vi "Data_taker_ver2.1.vi"() -> ()   [LabVIEW 2021]
uses:
  <vilib>/express/express analysis/Spectral/Block/exnSpectralBlock spectral measurements power poly.vi
  <vilib>/express/express analysis/Spectral/Block/exnSpectralBlock spectral measurements power DDT.vi
  <userlib>/SMC100 Controller_Drivers/SMC100.llb/enter / leave disable state.vi
  <vilib>/express/express analysis/Spectral/Block/exnSpectralBlock spectral measurements power WFM.vi
  <vilib>/express/express analysis/Spectral/XNode/ExpressSpectralMeasurementsBlockNode.xnode
panel:
  out "Loop count":i32
  in  "Averaging":bool
  out "Spectrum":cluster{"x axis":dbl[], "y data":dbl[]}(graph)
  out "Average intensity":cluster{"x axis":dbl[], "y data":dbl[]}(graph)
  out "Intensity (cut)":dynamicdata(graph)
  out "Spectrum":dynamicdata(graph)
  out "Intensity (raw)":dynamicdata(graph)
  in  "Repeat":i32
  out "Status":string
  in  "Begin Offset":dbl=1.0
  in  "Spectrum data path":path
  in  "Intensity data path":path
  in  "Velocity value (mm/s)":dbl
  in  "number of samples":i32=20000
  in  "rate":dbl=1000.0
  out "total time":dbl
  out "Displacement (mm)":dbl
  out "VISA Handle in":refnum<visa-resource-name>
  in  "unlock ?":bool
  in  "Unlock":bool
  out "Now position (mm)":dbl
  in  "Current absolute position":bool
  in  "Stop whole program":bool
  in  "Stop moving":bool
  in  "Start up/Reset":bool
  in  "Initialize":bool
  in  "Move  + data taking":bool
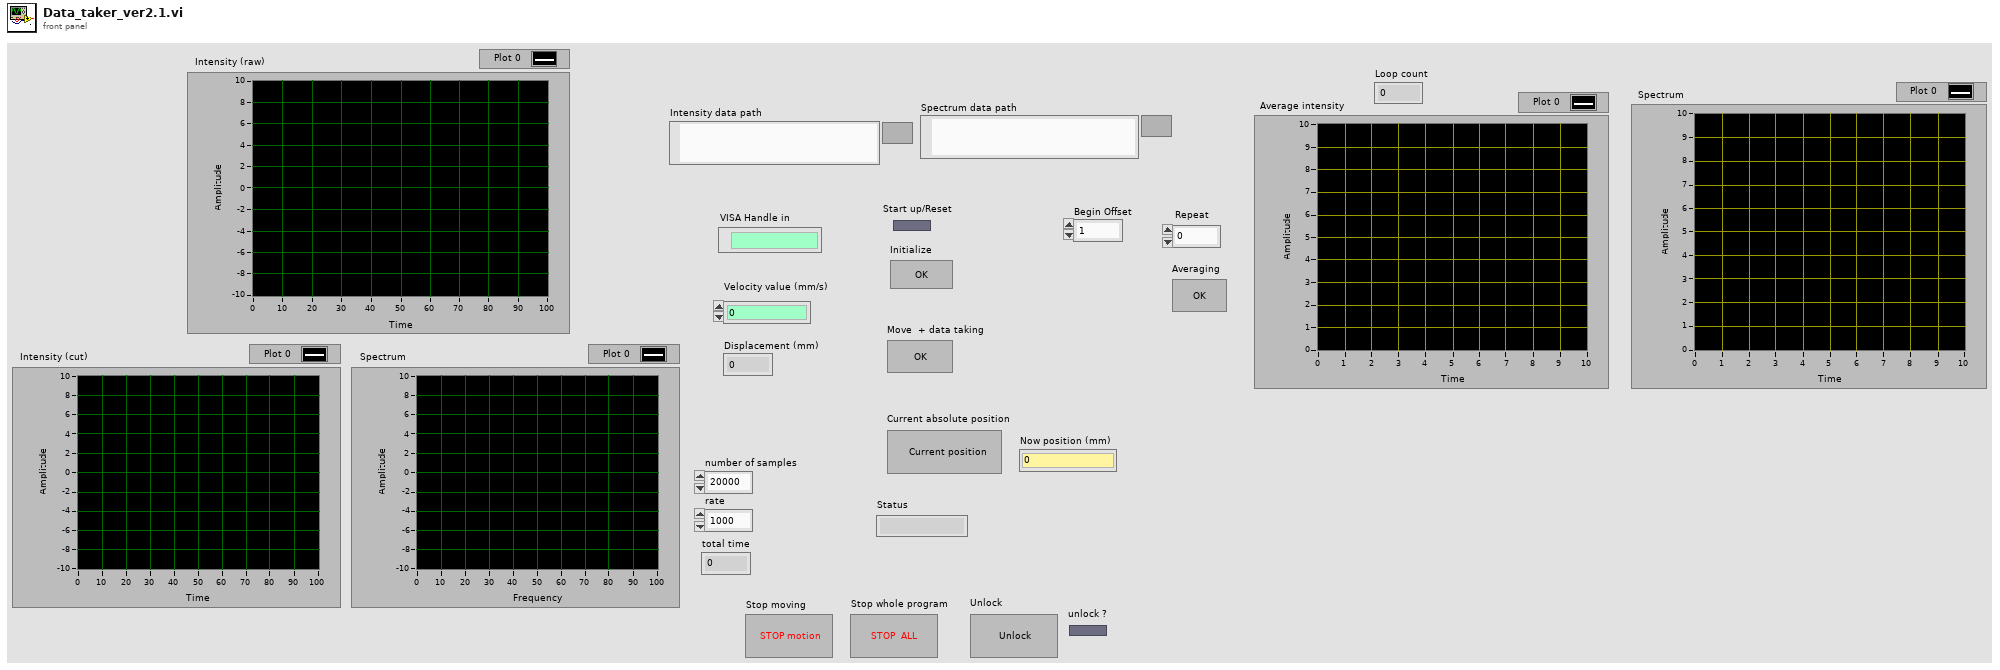
[diagram p1: front panel]
types:
  T1 = cluster{"averaging mode":u16, "weighting mode":u16, "number of averages":u32}
  T2 = cluster{"dB On (F)":bool, "unwrap phase (F)":bool, "convert to degree (F)":bool}
  T3 = enum16{"open", "replace", "create", "open or create", "replace or create", "replace or create with confirmation"}
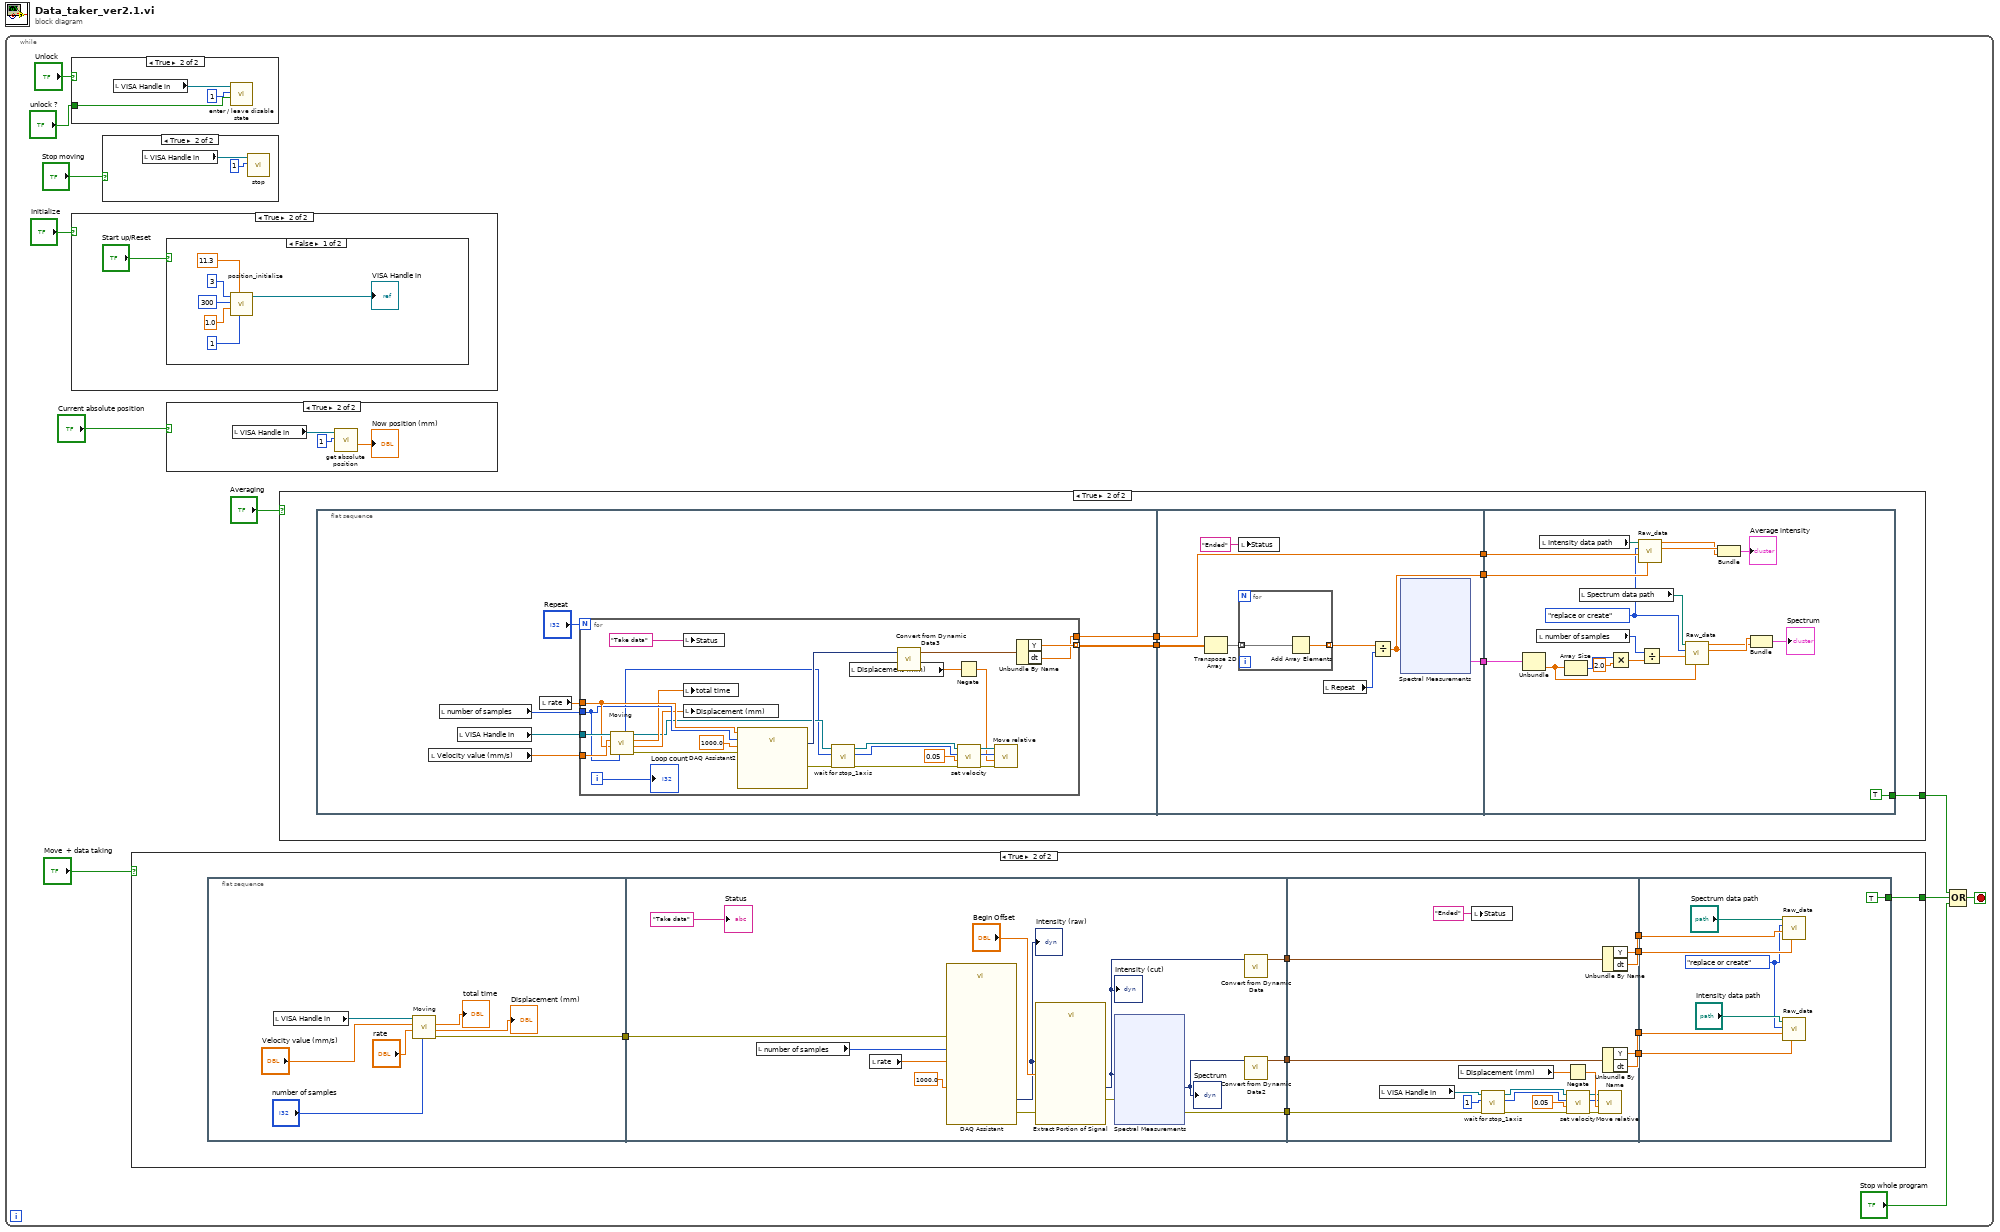
[diagram p0: block diagram]
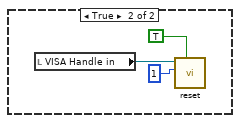
[diagram p8: hidden frame]
diagram:
  n1 = while {
    stop <- w2 stop-if-true
    n2 = case shown="True" "Unlock" {
      tunnel: "unlock ?" -> [_ w91]
      frame False {
      }
      frame True {
        n3 = local read "VISA Handle in"() -> (w90:refnum<visa-resource-name>)
        n4 = call "enter / leave disable state.vi"("enter disable state (True)"=w91, "Axis in"=1, "VISA handle in"=w90) -> ()  [unwired: 5 in, 4 out]
      }
    }
    n5 = case shown="True" "Initialize" {
      frame False {
      }
      frame True {
        n6 = case shown="False" "Start up/Reset" {
          frame False {
            n7 = call "position_initialize.vi"("Axis in"=1, "New target position (units)"=11.3, "Velocity value (units/s)"=1.0, "Timeout (ms)"=u32 300, "SerialPort"=u8 3) -> ("VISA Refnum out"=→"VISA Handle in":refnum<visa-resource-name>)  [unwired: 6 in]
          }
          frame True {
            n8 = local read "VISA Handle in"() -> (w172:refnum<visa-resource-name>)
            n9 = call <userlib>:"reset.vi"("Wait for Reset? (T)"=TRUE, "Axis in"=1, "VISA Handle in"=w172) -> ()  [unwired: 3 in, 4 out]
          }
        }
      }
    }
    n10 = case shown="True" "Stop moving" {
      frame False {
      }
      frame True {
        n11 = local read "VISA Handle in"() -> (w162:refnum<visa-resource-name>)
        n12 = call <userlib>:"stop.vi"("Axis in"=1, "VISA Handle in"=w162) -> ()  [unwired: 4 in, 4 out]
      }
    }
    n13 = case shown="True" "Move  + data taking" {
      tunnel: [_ w96] -> w4
      frame False {
      }
      frame True {
        n14 = flat-sequence {
          tunnel: [w104] -> w95
          tunnel: [w117] -> w99
          tunnel: [w116] -> w98
          tunnel: [w115] -> w97
          tunnel: w95 -> [w111]
          tunnel: [w135] -> w103
          tunnel: [w134] -> w102
          tunnel: [w137] -> w101
          tunnel: [w136] -> w100
          tunnel: w99 -> [w143]
          tunnel: w98 -> [w142]
          tunnel: w97 -> [w139]
          tunnel: w103 -> [w157]
          tunnel: w102 -> [w158]
          tunnel: w101 -> [w153]
          tunnel: w100 -> [w154]
          tunnel: [TRUE] -> w96
          frame #0 {
            n15 = local read "VISA Handle in"() -> (w110:refnum<visa-resource-name>)
            n16 = call "Moving.vi"("number of samples"="number of samples", "rate"="rate", "Velocity value (mm/s)"="Velocity value (mm/s)", "VISA Refnum in"=w110) -> ("error out"=w104:errorcluster, "Displacement"=→"Displacement (mm)":dbl, "Total time"=→"total time":dbl)  [unwired: 3 in, 2 out]
          }
          frame #1 {
            n17 = local read "number of samples"() -> (w123:i32)
            n18 = local read "rate"() -> (w124:dbl)
            n19 = call "DAQ Assistant"("rate"=w124, "number of samples"=w123, "timeout (s)"=1000.0, "error in"=w111) -> ("data"=w113:dynamicdata, "error out"=w120:errorcluster)  [unwired: 12 in, 2 out]
            "Intensity (raw)" <- w113
            n20 = call "Extract Portion of Signal"("error in (no error)"=w120, "Begin Offset"="Begin Offset", "Signals"=w113) -> ("error out"=w119:errorcluster, "Section"=w112:dynamicdata)  [unwired: 7 in]
            "Intensity (cut)" <- w112
            n21 = xnode "Spectral Measurements"("Signals"=w112, "error in (no error)"=w119) -> ("Power Spectrum"=w114:dynamicdata, "error out"=w115:errorcluster)
            "Spectrum" <- w114
            n22 = call "Convert from Dynamic Data"("Dynamic Data Type"=w112) -> ("Waveform"=w116:waveform(dbl))  [unwired: 3 in]
            n23 = call "Convert from Dynamic Data2"("Dynamic Data Type"=w114) -> ("Waveform"=w117:waveform(dbl))  [unwired: 3 in]
            "Status" <- "Take data"
          }
          frame #2 {
            n24 = local read "VISA Handle in"() -> (w150:refnum<visa-resource-name>)
            n25 = local read "Displacement (mm)"() -> (w151:dbl)
            n26 = local write "Status"("Ended") -> ()
            n27 = call <userlib>:"wait for stop_1axis.vi"("error in"=w139, "Axis in"=1, "VISA Handle in"=w150) -> ("error out"=w146:errorcluster, "Axis out"=w145:i32, "VISA Handle out"=w144:refnum<visa-resource-name>)  [unwired: 3 in, 1 out]
            n28 = Negate(x=w151) -> (-x=w152:dbl)
            n29 = call <userlib>:"set velocity.vi"("error in"=w146, "Velocity value (units/s)"=0.05, "Axis in"=w145, "VISA Handle in"=w144) -> ("error out"=w149:errorcluster, "Axis out"=w148:i32, "VISA Handle out"=w147:refnum<visa-resource-name>)  [unwired: 2 in, 1 out]
            n30 = call <userlib>:"Move relative.vi"("error in"=w149, "Displacement (units)"=w152, "Axis in"=w148, "VISA Handle in"=w147) -> ()  [unwired: 2 in, 4 out]
            n31 = Unbundle By Name(w142) -> ("Y"=w135:dbl[], "dt"=w134:dbl)
            n32 = Unbundle By Name(w143) -> ("Y"=w137:dbl[], "dt"=w136:dbl)
          }
          frame #3 {
            w155 = T3."replace or create" ("operation (0:open)")
            n33 = call "Raw_data.vi"("y axis"=w157, "dt/df"=w158, "operation (0:open)"=w155, "Data path"="Spectrum data path") -> ()  [unwired: 6 in, 2 out]
            n34 = call "Raw_data.vi"("y axis"=w153, "dt/df"=w154, "operation (0:open)"=w155, "Data path"="Intensity data path") -> ()  [unwired: 6 in, 2 out]
          }
        }
      }
    }
    n35 = case shown="True" "Current absolute position" {
      frame False {
      }
      frame True {
        n36 = local read "VISA Handle in"() -> (w93:refnum<visa-resource-name>)
        n37 = call <userlib>:"get absolute position.vi"("Axis in"=1, "VISA Handle in"=w93) -> ("Target position (units)"=→"Now position (mm)":dbl)  [unwired: 3 in, 4 out]
      }
    }
    n38 = case shown="True" "Averaging" {
      tunnel: [_ w15] -> w5
      frame False {
      }
      frame True {
        n39 = flat-sequence {
          tunnel: [w19] -> w17
          tunnel: [w18] -> w16
          tunnel: w17 -> [w54]
          tunnel: w16 -> [w52]
          tunnel: [w53] -> w14
          tunnel: [w52] -> w13
          tunnel: [w51] -> w12
          tunnel: [TRUE] -> w15
          tunnel: w14 -> [w77]
          tunnel: w13 -> [w76]
          tunnel: w12 -> [w74]
          frame #0 {
            n40 = local read "Velocity value (mm/s)"() -> (w20:dbl)
            n41 = local read "number of samples"() -> (w22:i32)
            n42 = local read "VISA Handle in"() -> (w23:refnum<visa-resource-name>)
            n43 = local read "rate"() -> (w21:dbl)
            n44 = for {
              N: "Repeat" -> [_]
              tunnel: w23 -> [w35]
              tunnel: w22 -> [w32]
              tunnel: w21 -> [w33]
              tunnel: w20 -> [w34]
              tunnel: [w48] -> w19 mode=indexing
              tunnel: [w26] -> w18
              i -> [w25]
              n45 = call "Moving.vi"("number of samples"=w32, "rate"=w33, "Velocity value (mm/s)"=w34, "VISA Refnum in"=w35) -> ("error out"=w31:errorcluster, "Displacement"=w30:dbl, "Total time"=w29:dbl, "VISA Refnum out"=w28:refnum<visa-resource-name>, "Axis out"=w27:i32)  [unwired: 3 in]
              n46 = local write "Status"("Take data") -> ()
              n47 = local write "total time"(w29) -> ()
              n48 = local write "Displacement (mm)"(w30) -> ()
              n49 = call "DAQ Assistant2"("rate"=w33, "number of samples"=w32, "timeout (s)"=1000.0, "error in"=w31) -> ("data"=w49:dynamicdata, "error out"=w50:errorcluster)  [unwired: 12 in, 2 out]
              n50 = call <userlib>:"wait for stop_1axis.vi"("error in"=w50, "Axis in"=w27, "VISA Handle in"=w28) -> ("error out"=w39:errorcluster, "Axis out"=w40:i32, "VISA Handle out"=w41:refnum<visa-resource-name>)  [unwired: 3 in, 1 out]
              n51 = local read "Displacement (mm)"() -> (w38:dbl)
              n52 = call "Convert from Dynamic Data3"("Dynamic Data Type"=w49) -> ("Waveform"=w36:waveform(dbl))  [unwired: 3 in]
              n53 = Negate(x=w38) -> (-x=w37:dbl)
              n54 = call <userlib>:"set velocity.vi"("error in"=w39, "Velocity value (units/s)"=0.05, "Axis in"=w40, "VISA Handle in"=w41) -> ("error out"=w45:errorcluster, "Axis out"=w44:i32, "VISA Handle out"=w43:refnum<visa-resource-name>)  [unwired: 2 in, 1 out]
              n55 = call <userlib>:"Move relative.vi"("error in"=w45, "Displacement (units)"=w37, "Axis in"=w44, "VISA Handle in"=w43) -> ()  [unwired: 2 in, 4 out]
              n56 = Unbundle By Name(w36) -> ("Y"=w48:dbl[], "dt"=w26:dbl)
              "Loop count" <- w25
            }
          }
          frame #1 {
            n57 = Transpose 2D Array(2D array=w54) -> (transposed array=w56:dbl[][])
            n58 = local write "Status"("Ended") -> ()
            n59 = for {
              tunnel: w56 -> [w69] mode=indexing
              tunnel: [w68] -> w57 mode=indexing
              n60 = Add Array Elements(numeric array=w69) -> (sum=w68:dbl)
            }
            n61 = local read "Repeat"() -> (w58:i32)
            n62 = Divide(x=w57, y=w58) -> (x/y=w53:dbl[])
            n63 = xnode "Spectral Measurements"("Signals"=w53) -> ("Power Spectrum"=w51:cluster{"f0":dbl, "df":dbl, "magnitude":dbl[]})  [unwired: 1 in, 1 out]
          }
          frame #2 {
            w75 = T3."replace or create" ("operation (0:open)")
            n64 = Unbundle(w74) -> ("magnitude"=w84:dbl[])  [unwired: 2 out]
            n65 = local read "number of samples"() -> (w81:i32)
            n66 = local read "Intensity data path"() -> (w80:path)
            n67 = Array Size(array=w84) -> (size(s)=w85:i32)
            n68 = local read "Spectrum data path"() -> (w79:path)
            n69 = Multiply(x=w85, y=2.0) -> (x*y=w82:dbl)
            n70 = call "Raw_data.vi"("y axis"=w77, "dt/df"=w76, "operation (0:open)"=w75, "Data path"=w80) -> ("x axis"=w73:dbl[], "y data"=w72:dbl[])  [unwired: 6 in]
            n71 = Divide(x=w81, y=w82) -> (x/y=w83:dbl)
            n72 = call "Raw_data.vi"("y axis"=w84, "dt/df"=w83, "operation (0:open)"=w75, "Data path"=w79) -> ("x axis"=w71:dbl[], "y data"=w70:dbl[])  [unwired: 6 in]
            n73 = Bundle("x axis"=w73, "y data"=w72) -> (→"Average intensity":cluster{"x axis":dbl[], "y data":dbl[]})  [unwired: 1 in]
            n74 = Bundle("x axis"=w71, "y data"=w70) -> (→"Spectrum":cluster{"x axis":dbl[], "y data":dbl[]})  [unwired: 1 in]
          }
        }
      }
    }
    n75 = Compound Arithmetic op=OR(w5, w4, "Stop whole program") -> (w2:bool)
  }
